vi "FlatToRichcif_plugincore_Error.vi"(5 "OutputClusterType":T1, 11 "InputCluster":T2) -> (3 "OutputCluster":T1)   [LabVIEW 2021, in "CIF_Launcher_client.lvlib"]
uses:
  CIF_Launcher_client.lvlib
  cif_plugincore_Error_Flat.ctl
  cif_plugincore_Error.ctl
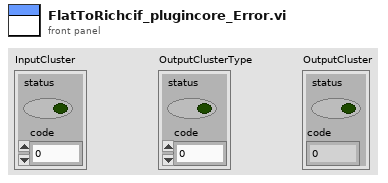
[diagram p1: front panel]
types:
  T1 = typedef "CIF_Launcher_client.lvlib/cif_plugincore_Error.ctl" = cluster{"status":bool, "code":i32}
  T2 = typedef "CIF_Launcher_client.lvlib/cif_plugincore_Error_Flat.ctl" = cluster{"status":bool, "code":i32}
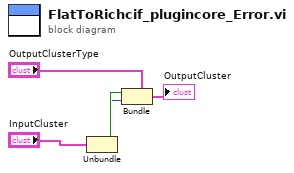
[diagram p0: block diagram]
diagram:
  n1 = Unbundle "Unbundle"("InputCluster") -> ("status"=w2:bool, "code"=w1:i32)
  n2 = Bundle "Bundle"(cluster="OutputClusterType", "status"=w2, "code"=w1) -> (→"OutputCluster":T1)
